vi "Write Key-Value.vi"(8 "Error In":errorcluster, 10 "Pair":cluster{"Key":string, "Value":string}, 11 "String in":refnum<class "String.lvclass">) -> (0 "Error Out":errorcluster, 3 "String out":refnum<class "String.lvclass">)   [LabVIEW 2018, in "Toolkit.lvlib" / "Loaders.lvlib" / "String.lvclass"]
doc: "Adds a new key-value pair, where the value is a string that contains a partial Mustache template."
uses:
  String.lvclass
  String.lvclass/String.ctl
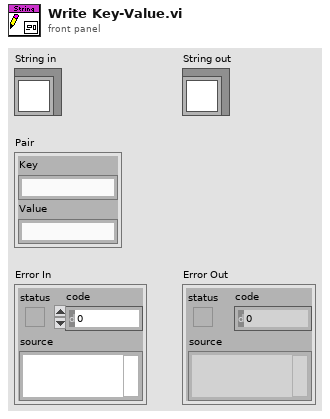
[diagram p1: front panel]
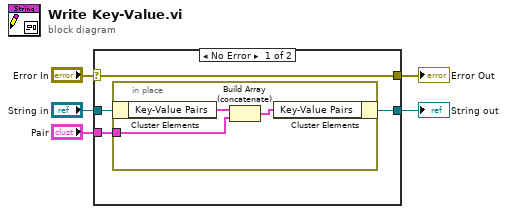
[diagram p0: block diagram]
diagram:
  n1 = case shown="No Error" "Error In" {
    selector: "Error In" -> [w9 w14]
    tunnel: [w9 w14] -> w4
    tunnel: [w7 w13] -> w2
    tunnel: "String in" -> [w8 w13]
    tunnel: "Pair" -> [w6 _]
    frame No Error {
      n2 = in-place {
        in-place-border: w6 -> [w10]
        n3 = in-place-cluster #1(w8) -> ("Key-Value Pairs"=w12:cluster{"Key":string, "Value":string}[])
        n4 = Build Array (concatenate)(w12, w10) -> (w11:cluster{"Key":string, "Value":string}[])
        n5 = in-place-cluster #1("Key-Value Pairs"=w11) -> (w7:refnum<class "String.lvclass">)
      }
    }
    frame Error {
    }
  }
  "Error Out" <- w4
  "String out" <- w2
